vi "prueba.vi"(7 "error in":errorcluster) -> (20 "Image Out":T9(plugin-control), 22 "Tokenized Output Data":T2(array[cluster]) {"Stream Mode" items=["Numeric", "AlphaNumeric", "Raw Bytes", "UCC/EAN-128 - In Tokens", "UCC/EAN-128 - In Data", "Extended Character Interpretation", "Kanji"]}, 24 "QR Code Report":T3={"Found?"=FALSE, "Data"="", "Bounding Box"=[], "Errors Corrected"=0, "Dimensions (Rows/Cols)"=0, "Version"=0, "QR Model"=0, "Stream Mode"=0, "Barcode Polarity"=-2, "Mirrored?"=FALSE, "Append Stream Position"=0, "Size of Append Stream"=0, "First EAN-128 ID"=0, "First Alternate Language ID"=0, "Append Stream ID"=0, "Minimum Edge Strength"=30, "Demodulation Mode"=-2, "Cell Sample Size"=-2, "Cell Filter Mode"=-2} {"Append Stream ID" format="%x"; "Cell Filter Mode" items=["Auto-detect"=-2, "Average"=0, "Median"=1, "Central Average"=2, "High Average"=3, "Low Average"=4, "Very High Average"=5, "Very Low Average"=6, "All Filters"=8]; "Cell Sample Size" items=["Auto-detect"=-2, "1x1"=1, "2x2"=2, "3x3"=3, "4x4"=4, "5x5"=5, "6x6"=6, "7x7"=7]; "Demodulation Mode" items=["Auto-detect"=-2, "Histogram"=0, "Local Contrast"=1, "Combination"=2, "All"=3]; "Barcode Polarity" items=["Auto-detect"=-2, "Black on White"=0, "White on Black"=1]; "Stream Mode" items=["Numeric", "AlphaNumeric", "Raw Bytes", "UCC/EAN-128 - In Tokens", "UCC/EAN-128 - In Data", "Extended Character Interpretation", "Kanji"]; "QR Model" items=["Auto-detect", "Micro", "Model 1", "Model 2"]; "Version" max=40 step=1}, 27 "error out":errorcluster)   [LabVIEW 2018]
uses:
  <vilib>/vision/Instrument.llb/QR Code Report.ctl
  <vilib>/vision/Instrument.llb/QR Code Model Type.ctl
  <vilib>/vision/Instrument.llb/QR Code Stream Mode Type.ctl
  <vilib>/vision/Instrument.llb/Data Matrix Polarity.ctl
  <vilib>/vision/Instrument.llb/Demodulation Mode.ctl
  <vilib>/vision/Instrument.llb/Cell Sample Size.ctl
  <vilib>/vision/Instrument.llb/Cell Filter Mode.ctl
  <vilib>/vision/NI_Vision_Development_Module.lvlib
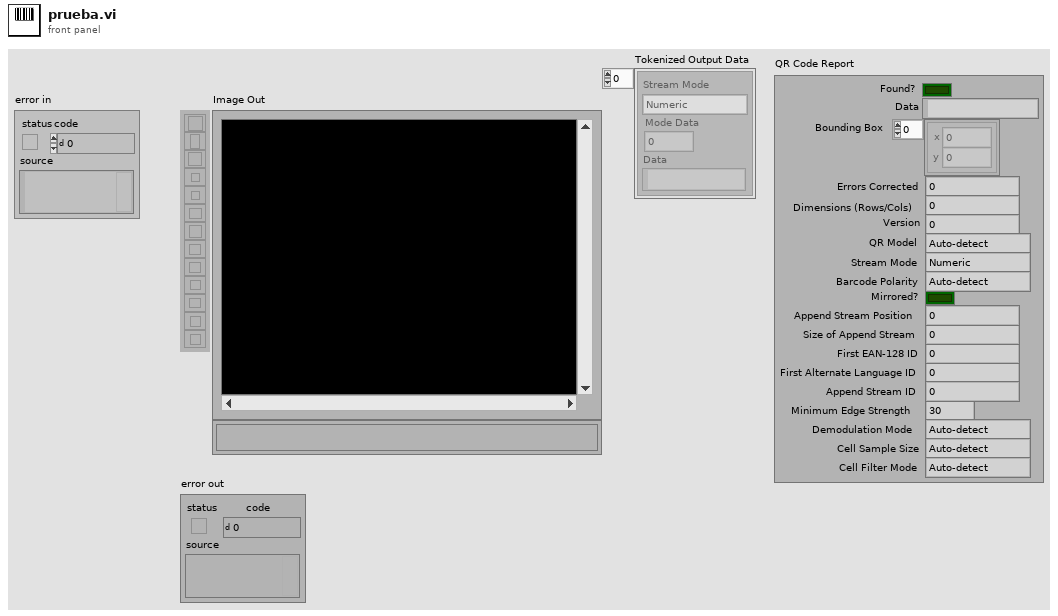
[diagram p1: front panel]
types:
  T1 = typedef "QR Code Stream Mode Type.ctl" = i32
  T2 = cluster{"Stream Mode":T1, "Mode Data":u32, "Data":string}[]
  T3 = typedef "QR Code Report.ctl" = cluster{"Found?":bool, "Data":string, "Bounding Box":cluster{"x":sgl, "y":sgl}[], "Errors Corrected":u32, "Dimensions (Rows/Cols)":u32, "Version":u32, "QR Model":T4, "Stream Mode":T1, "Barcode Polarity":T5, "Mirrored?":bool, "Append Stream Position":u32, "Size of Append Stream":u32, "First EAN-128 ID":i32, "First Alternate Language ID":i32, "Append Stream ID":u32, "Minimum Edge Strength":u32, "Demodulation Mode":T6, "Cell Sample Size":T7, "Cell Filter Mode":T8}
  T4 = typedef "QR Code Model Type.ctl" = i32
  T5 = typedef "Data Matrix Polarity.ctl" = i32
  T6 = typedef "Demodulation Mode.ctl" = i32
  T7 = typedef "Cell Sample Size.ctl" = i32
  T8 = typedef "Cell Filter Mode.ctl" = i32
  T9 = typedef "IMAQ Image.ctl" = refnum<image>
  T10 = cluster{"Matrix Dimensions (cells)":i32, "Barcode Polarity":i32, "Mirror Mode":i32, "QR Model":i32}
  T11 = cluster{"Rotation Mode":enum32{"Unlimited", "0 Degrees", "90 Degrees", "180 Degrees", "270 Degrees"}, "Skip Location?":bool, "Edge Threshold":u32, "Demodulation Mode":i32, "Cell Sample Size":i32, "Cell Filter Mode":i32, "Skew Degrees Allowed":u32}
  T12 = cluster{"Global Rectangle":i32[], "Contours":cluster{"ID":enum32{"External", "Internal"}, "Type":u32, "Coordinates":i32[]}[]}
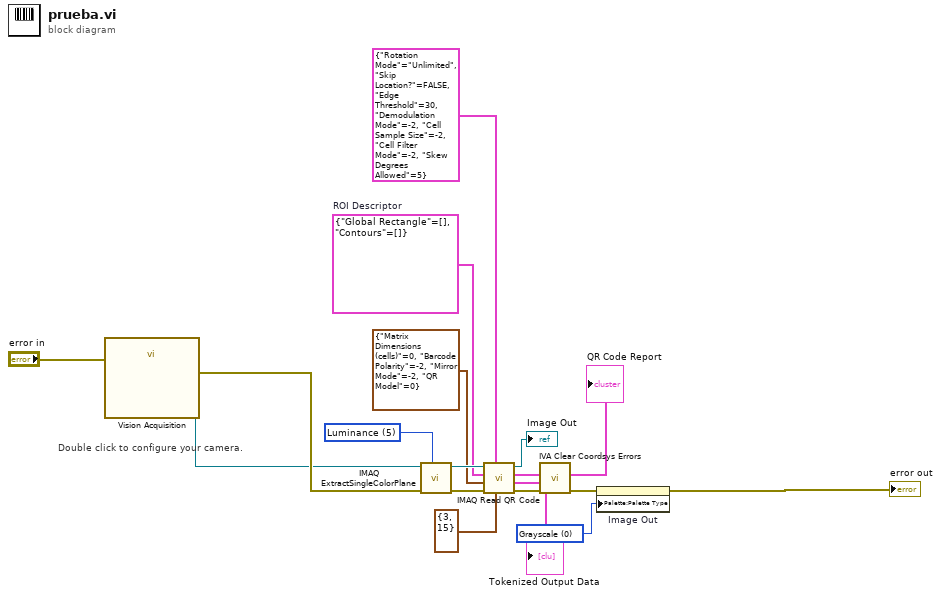
[diagram p0: block diagram]
diagram:
  w4 = u32 0 items=["Grayscale", "Binary", "Gradient", "Rainbow", "Temperature", "User Defined", "Binary 16 Bit", "Gradient 16 Bit", "Rainbow 16 Bit", "Temperature 16 Bit", "User Defined 16 Bit"] ("Palette Type")
  w10 = T12 {"Global Rectangle"=[], "Contours"=[]}  # ROI Descriptor
  w16 = 5 items=["Red", "Green", "Blue", "Hue", "Saturation", "Luminance", "Value", "Intensity"] ("Color Plane")
  # "Double click to configure your camera."
  n1 = call "Vision Acquisition"("error in"="error in") -> ("Image Out"=w1:T9, "error out"=w15:errorcluster)  [unwired: 24 in, 1 out]
  n2 = call "IMAQ ExtractSingleColorPlane"("Color Plane"=w16, "error in (no error)"=w15, "Image Src"=w1) -> ("error out"=w9:errorcluster, "Image Dst Out"=w14:T9)  [unwired: 1 in, 6 out]
  n3 = call "IMAQ Read QR Code"("QR Code Cell Size (pixels)"=cluster{"Minimum Size":u32, "Maximum Size":u32} {"Minimum Size"=3, "Maximum Size"=15}, "QR Search Options"=T11 {"Rotation Mode"=enum."Unlimited", "Skip Location?"=FALSE, "Edge Threshold"=30, "Demodulation Mode"=-2, "Cell Sample Size"=-2, "Cell Filter Mode"=-2, "Skew Degrees Allowed"=5}, "error in (no error)"=w9, "QR Description Options"=T10 {"Matrix Dimensions (cells)"=0, "Barcode Polarity"=-2, "Mirror Mode"=-2, "QR Model"=0}, "ROI Descriptor"=w10, "Image"=w14) -> ("error out"=w8:errorcluster, "Tokenized Output Data"=→"Tokenized Output Data":T2, "QR Code Report"=→"QR Code Report":T3, "Image (duplicate)"=→"Image Out":T9)  [unwired: 1 in, 1 out]
  n4 = call <vilib>:"IVA Clear Coordsys Errors.vi"("error in (no error)"=w8) -> ("error out"=w7:errorcluster)  [unwired: 10 in]
  n5 = property on="Image Out" class="ImageControl"(error in=w7, "Palette:Palette Type"=w4) -> (error out=→"error out":errorcluster)  [unwired: 1 in, 1 out]
